vi "TextFit_Find Next Priority and Shrink.vi"(7 "Font Size":T3=enum."Thin", 8 "Error":errorcluster, 9 "Do Not Shrink":bool, 10 "Reset Prioity":bool, 11 "Array":T1[](array[typedef])) -> (0 "Error Out":errorcluster, 2 "All Items Shrunk Out":bool, 3 "Array Out":T1[](array[typedef]))   [LabVIEW 2014]
doc: "Finds the next letter in the Character array to be compressed and compresses it"
uses:
  Controls/Cluster/Cluster_Character Size and Priority Data.ctl
  Controls/String_Picture/String Char Normal.ctl
  Controls/Enum/ENUM_Font Size Select.ctl
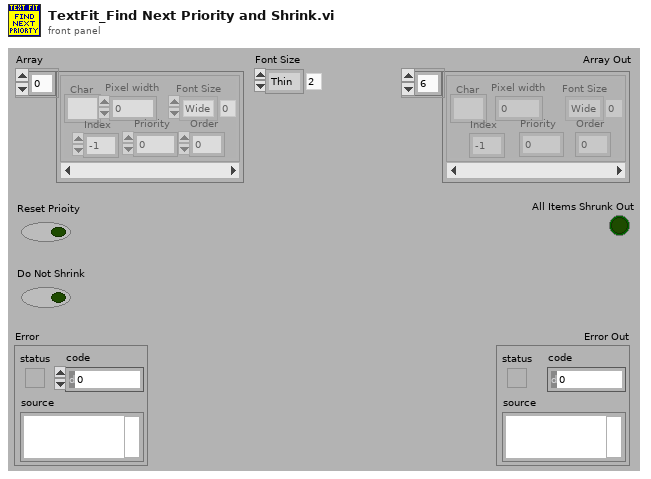
[diagram p1: front panel]
types:
  T1 = typedef "Cluster_Character Size and Priority Data.ctl" = cluster{"Char":T2, "Font Size":T3, "Pixel width":i32, "Priority":i32, "Order":i32, "Index":i32}
  T2 = typedef "String Char Normal.ctl" = string
  T3 = typedef "ENUM_Font Size Select.ctl" = enum16{"Wide", "Med", "Thin"}
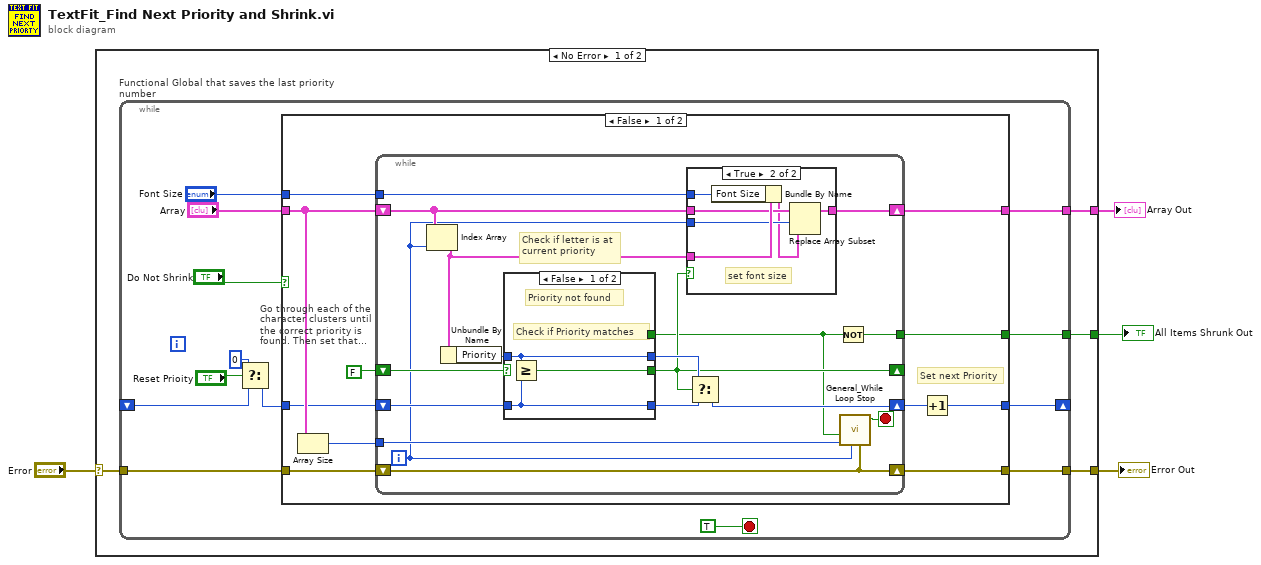
[diagram p0: block diagram]
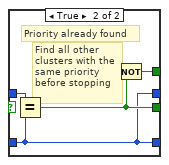
[diagram p2: hidden frame]
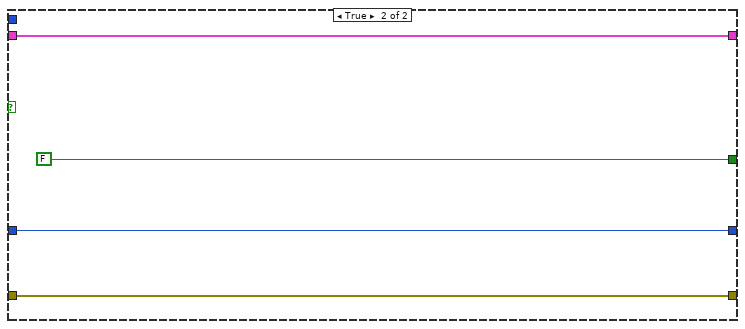
[diagram p4: hidden frame]
diagram:
  n1 = case shown="No Error" "Error" {
    selector: "Error" -> [w7 w68]
    tunnel: [w8 w68] -> w4
    tunnel: [w6 _] -> w2
    tunnel: [w5 _] -> w1
    frame No Error {
      n2 = while "Functional Global that saves the last priority number" {
        shift-right: [w11] -> _
        shift-left: _ -> [w17]
        tunnel: w7 -> [w14]
        tunnel: [w13] -> w8
        tunnel: [w12] -> w6
        tunnel: [w9] -> w5
        stop <- TRUE stop-if-true
        n3 = Select(t=0, s="Reset Prioity", f=w17) -> (s? t:f=w16:i32)
        n4 = case shown="False" "Do Not Shrink" {
          tunnel: "Font Size" -> [w32 _]
          tunnel: "Array" -> [w31 w67]
          tunnel: w16 -> [w29 w66]
          tunnel: w14 -> [w28 w65]
          tunnel: [w27 w65] -> w13
          tunnel: [w26 w67] -> w12
          tunnel: [w24 w66] -> w11
          tunnel: [w23 FALSE] -> w9
          frame False {
            # "Set next Priority"
            n5 = Array Size(array=w31) -> (size(s)=w22:i32)
            n6 = while "Go through each of the character clusters until the correct priority is found. Then set that cluster to the current\nfont size." {
              shift-right: [w42] -> w27
              shift-left: w28 -> [w42]
              shift-right: [w46] -> w26
              shift-left: w31 -> [w47]
              tunnel: w32 -> [w49]
              tunnel: w22 -> [w36]
              shift-right: [w39] -> _
              shift-left: FALSE -> [w44]
              shift-right: [w40] -> w25
              shift-left: w29 -> [w38]
              tunnel: [w33] -> w23
              i -> [w35]
              stop <- w43 stop-if-true
              # "Check if letter is at\ncurrent priority"
              n7 = Index Array(array=w47, index=w35) -> (element=w48:T1)
              n8 = Unbundle By Name(w48) -> ("Priority"=w45:i32)
              n9 = case shown="False" w44 {
                tunnel: w38 -> [w50 w53]
                tunnel: [w52 w55] -> w39
                tunnel: w45 -> [w51 w56]
                tunnel: [_ w54] -> w34
                tunnel: [w51 w53] -> w41
                tunnel: [w50 w53] -> w37
                frame False {
                  # "Check if Priority matches"
                  # "Priority not found"
                  n10 = Greater Or Equal?(x=w51, y=w50) -> (x >= y?=w52:bool)
                }
                frame True {
                  # "Find all other \nclusters with the\nsame priority\nbefore stopping"
                  # "Priority already found"
                  n11 = Equal?(x=w56, y=w53) -> (x = y?=w55:bool)
                  n12 = Not(x=w55) -> (.not. x?=w54:bool)
                }
              }
              n13 = case shown="True" w39 {
                tunnel: w49 -> [_ w60]
                tunnel: w48 -> [_ w63]
                tunnel: w47 -> [w57 w62]
                tunnel: [w57 w61] -> w46
                tunnel: w35 -> [_ w59]
                frame False {
                }
                frame True {
                  # "set font size"
                  n14 = Bundle By Name(cluster=w63, "Font Size"=w60) -> (w58:T1)
                  n15 = Replace Array Subset(array=w62, new element=w58, index=w59) -> (w61:T1[])
                }
              }
              n16 = Select(t=w41, s=w39, f=w37) -> (s? t:f=w40:i32)
              n17 = Not(x=w34) -> (.not. x?=w33:bool)
              n18 = call "General_While Loop Stop.vi"("Error In"=w42, "Index In"=w35, "Array Size In"=w36, "Stop 3 In"=w34) -> ("Stop Out1"=w43:bool)  [unwired: 3 in, 3 out]
            }
            n19 = Increment(x=w25) -> (x+1=w24:i32)
          }
          frame True {
          }
        }
      }
    }
    frame Error {
    }
  }
  "Error Out" <- w4
  "All Items Shrunk Out" <- w1
  "Array Out" <- w2
